vi "Auto Left Right Drive.vi"(9 "Right":dbl=125.0, 10 "Left":dbl=125.0, 11 "Run?":bool) -> (3 "Done":bool)   [LabVIEW 2013]
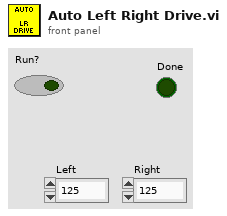
[diagram p1: front panel]
types:
  T1 = typedef "WPI_EncoderDevRef.ctl" = cluster{"DevStatus":errorcluster, "EncoderIndex":T2, "CounterIndex":T3, "DistancePerCount":dbl, "Decoding Type":T4}
  T2 = typedef "FPGA_EncoderIdx.ctl" = enum8{"Enc 0", "Enc 1", "Enc 2", "Enc 3", "Invalid"}
  T3 = typedef "FPGA_CounterCtrSystemIndex.ctl" = enum8{"Ctr 0", "Ctr 1", "Ctr 2", "Ctr 3", "Ctr 4", "Ctr 5", "Ctr 6", "Ctr 7", "Invalid"}
  T4 = typedef "WPI_EncoderType.ctl" = enum16{"1x", "2x", "4x"}
  T5 = typedef "WPI_MotorControlDeviceRef.ctl" = cluster{"DeviceStatus":errorcluster, "Type":enum16{"PWM", "CAN"}, "PWM":cluster{"Digital Module":T6, "PWM Channel":T7, "DeadBand":T8}, "CAN":cluster{"Device Number":u8, "Control Mode":T9, "Semaphore":T10, "Max Vout":dbl}, "Invert":bool, "TransformRef":T11, "InvTransformRef":T11}
  T6 = typedef "FPGA_TypedefDigitalModule.ctl" = enum16{"Digital Module 1", "Digital Module 2"}
  T7 = typedef "FPGA_DIOPWMChannel.ctl" = enum8{"PWM 1", "PWM 2", "PWM 3", "PWM 4", "PWM 5", "PWM 6", "PWM 7", "PWM 8", "PWM 9", "PWM 10", "Invalid"}
  T8 = typedef "WPI_PWMDeadband.ctl" = cluster{"Name":string, "maxPositivePwm":i32, "minPositivePwm":i32, "centerPwm":i32, "maxNegativePwm":i32, "minNegativePwm":i32, "angularRange":u16}
  T9 = typedef "WPI_CANJaguar_ControlMode.ctl" = enum8{"Percent VBus", "Current", "Speed", "Position", "Voltage"}
  T10 = typedef "Semaphore RefNum" = refnum<k1>
  T11 = typedef "WPI_PWMTransform_ConPane.ctl" = refnum<vi>
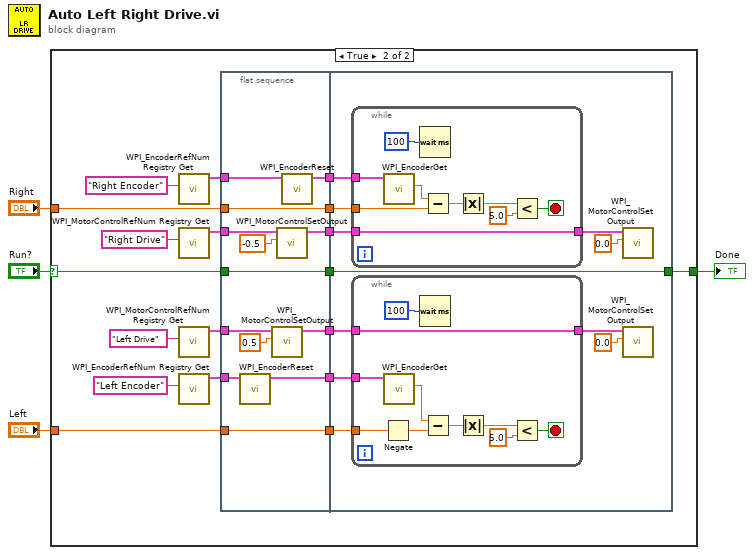
[diagram p0: block diagram]
diagram:
  n1 = case shown="True" "Run?" {
    selector: "Run?" -> [w5 w10]
    tunnel: [w5 w9] -> w3
    tunnel: "Left" -> [_ w11]
    tunnel: "Right" -> [_ w6]
    frame False {
    }
    frame True {
      n2 = call <vilib>:"WPI_EncoderRefNum Registry Get.vi"("refnum name"="Right Encoder") -> ("EncoderDevRef"=w18:T1)  [unwired: 9 in, 1 out]
      n3 = call <vilib>:"WPI_MotorControlRefNum Registry Get.vi"("refnum name"="Right Drive") -> ("MotorControlDevRef"=w16:T5)  [unwired: 9 in, 1 out]
      n4 = call <vilib>:"WPI_MotorControlRefNum Registry Get.vi"("refnum name"="Left Drive") -> ("MotorControlDevRef"=w13:T5)  [unwired: 9 in, 1 out]
      n5 = call <vilib>:"WPI_EncoderRefNum Registry Get.vi"("refnum name"="Left Encoder") -> ("EncoderDevRef"=w20:T1)  [unwired: 9 in, 1 out]
      n6 = flat-sequence {
        tunnel: w13 -> [w37]
        tunnel: w16 -> [w34]
        tunnel: [w33] -> w24
        tunnel: [w32] -> w23
        tunnel: [w28] -> w22
        tunnel: w18 -> [w29]
        tunnel: [w30] -> w21
        tunnel: w20 -> [w31]
        tunnel: [w27] -> w12
        tunnel: w11 -> [w27]
        tunnel: w10 -> [w26]
        tunnel: [w26] -> w8
        tunnel: [w25] -> w7
        tunnel: w6 -> [w25]
        tunnel: w24 -> [w46]
        tunnel: w23 -> [w45]
        tunnel: w22 -> [w48]
        tunnel: w21 -> [w47]
        tunnel: w12 -> [w40]
        tunnel: [w39] -> w9
        tunnel: w8 -> [w39]
        tunnel: w7 -> [w38]
        frame #0 {
          n7 = call <vilib>:"WPI_EncoderReset.vi"("EncoderDevRef"=w31) -> ("EncoderDevRef"=w30:T1)  [unwired: 9 in, 1 out]
          n8 = call <vilib>:"WPI_MotorControlSetOutput.vi"("Output"=0.5, "MotorControlDevRef"=w37) -> ("MotorControlDevRef"=w33:T5)  [unwired: 7 in, 2 out]
          n9 = call <vilib>:"WPI_MotorControlSetOutput.vi"("Output"=-0.5, "MotorControlDevRef"=w34) -> ("MotorControlDevRef"=w32:T5)  [unwired: 7 in, 2 out]
          n10 = call <vilib>:"WPI_EncoderReset.vi"("EncoderDevRef"=w29) -> ("EncoderDevRef"=w28:T1)  [unwired: 9 in, 1 out]
        }
        frame #1 {
          n11 = while {
            tunnel: w48 -> [w66]
            tunnel: [w65] -> w44
            tunnel: w45 -> [w65]
            tunnel: w38 -> [w59]
            stop <- w60 stop-if-true
            n12 = call <vilib>:"WPI_EncoderGet.vi"("EncoderDevRef"=w66) -> ("Distance"=w64:dbl)  [unwired: 5 in, 5 out]
            n13 = Wait (ms)(milliseconds to wait=u32 100) -> ()  [unwired: 1 out]
            n14 = Subtract(x=w64, y=w59) -> (x-y=w63:dbl)
            n15 = Absolute Value(x=w63) -> (abs(x)=w62:dbl)
            n16 = Less?(x=w62, y=5.0) -> (x < y?=w60:bool)
          }
          n17 = while {
            tunnel: w47 -> [w57]
            tunnel: w46 -> [w56]
            tunnel: [w56] -> w42
            tunnel: w40 -> [w50]
            stop <- w51 stop-if-true
            n18 = Negate(x=w50) -> (-x=w49:dbl)
            n19 = call <vilib>:"WPI_EncoderGet.vi"("EncoderDevRef"=w57) -> ("Distance"=w52:dbl)  [unwired: 5 in, 5 out]
            n20 = Wait (ms)(milliseconds to wait=u32 100) -> ()  [unwired: 1 out]
            n21 = Subtract(x=w52, y=w49) -> (x-y=w54:dbl)
            n22 = Absolute Value(x=w54) -> (abs(x)=w53:dbl)
            n23 = Less?(x=w53, y=5.0) -> (x < y?=w51:bool)
          }
          n24 = call <vilib>:"WPI_MotorControlSetOutput.vi"("Output"=0.0, "MotorControlDevRef"=w44) -> ()  [unwired: 7 in, 3 out]
          n25 = call <vilib>:"WPI_MotorControlSetOutput.vi"("Output"=0.0, "MotorControlDevRef"=w42) -> ()  [unwired: 7 in, 3 out]
        }
      }
    }
  }
  "Done" <- w3
